vi "Voltage - Continuous Input_0317.vi"() -> ()   [LabVIEW 2021]
doc: "This example demonstrates how to continuously acquire buffered voltage measurements using a DAQmx device.\n\nFor instructions on how to connect your signals to the DAQ device, refer to your device documentation."
uses:
  <vilib>/Utility/error.llb/DialogType.ctl
  <vilib>/DAQmx/read.llb/DAQmx Read (Analog 1D Wfm NChan NSamp).vi
  <vilib>/DAQmx/create/channels.llb/DAQmx Create Channel (AI-Voltage-Basic).vi
  <vilib>/DAQmx/configure/timing.llb/DAQmx Timing (Sample Clock).vi
  <vilib>/DAQmx/configure/task.llb/DAQmx Configure Logging (TDMS).vi
  <vilib>/DAQmx/configure/trigger.llb/DAQmx Start Trigger (Digital Edge).vi
  <vilib>/DAQmx/configure/trigger.llb/DAQmx Start Trigger (Time).vi
  <vilib>/DAQmx/configure/trigger.llb/DAQmx Start Trigger (Analog Edge).vi
  <vilib>/DAQmx/miscellaneous.llb/DAQmx Fill In Error Info.vi
  <resource>/objmgr/daqmx.rc
panel:
  in  "Physical Channel 2":tag="Dev1/ai0"
  in  "Min Voltage 2":dbl=-5.0
  in  "Max Voltage 2":dbl=5.0
  in  "Trigger Type":T1(tab)
  in  "Digital Start Trigger Edge":i32(ring)=10280 caption="Edge" items=["Rising"=10280, "Falling"=10171]
  in  "Digital Start Trigger Source":tag="/Dev1/PFI0" caption="Source"
  in  "Digital Pause Trigger Pause When":i32(ring)=10192 caption="Pause When" items=["High"=10192, "Low"=10214]
  in  "Digital Pause Trigger Source":tag="/Dev1/PFI0" caption="Source"
  in  "Analog Start Trigger Level":dbl caption="Level" format="%0.2f"
  in  "Analog Start Trigger Hysteresis":dbl caption="Hysteresis" format="%.2f"
  in  "Analog Start Trigger Slope":i32(ring)=10280 caption="Slope" items=["Rising"=10280, "Falling"=10171]
  in  "Analog Start Trigger Source":string="APFI0" caption="Source"
  in  "Analog Pause Trigger Source":string="APFI0" caption="Source"
  in  "Analog Pause Trigger Pause When":i32(ring)=10093 caption="Pause When" items=["Above Level"=10093, "Below Level"=10107]
  in  "Analog Pause Trigger Level":dbl caption="Level" format="%.2f"
  in  "When":timestamp
  in  "Select Time\nManually":bool
  in  "Stop":bool
  out "Waveform Graph":waveform(dbl)[](graph)
  in  "TDMS File Path":path
  in  "Number of Samples":i32=100
  in  "Sample Rate":dbl=1000.0
  in  "Sample Clock Source":tag="OnboardClock"
  in  "Terminal Configuration":i32(ring)=-1 items=["default"=-1, "RSE"=10083, "NRSE"=10078, "Differential"=10106, "Pseudodifferential"=12529]
  in  "Max Voltage":dbl=5.0
  in  "Min Voltage":dbl=-5.0
  in  "Physical Channel":tag="Dev1/ai0"
  out "Actual Sample Rate":dbl=1000.0 format="%0.2f"
  in  "Logging Mode":i32(ring)=10231 items=["Off"=10231, "Log and Read"=15842]
  # "Channel Settings"
  # "Acquired Data"
  # "Timing Settings"
  # "Trigger Settings"
  # "Logging Settings"
  # "To enable triggers, select a tab above, and configure the settings.\n\nNot all hardware supports all trigger types. Refer to your device documentation for more information."
  # "This trigger type is not supported in continuous sample timing. \n\nRefer to your device documentation for more information on which triggers are supported."
  # "This trigger type is not supported in continuous sample timing. \n\nRefer to your device documentation for more information on which triggers are supported."
  # "If time is not manually set, task will begin after 10 seconds"
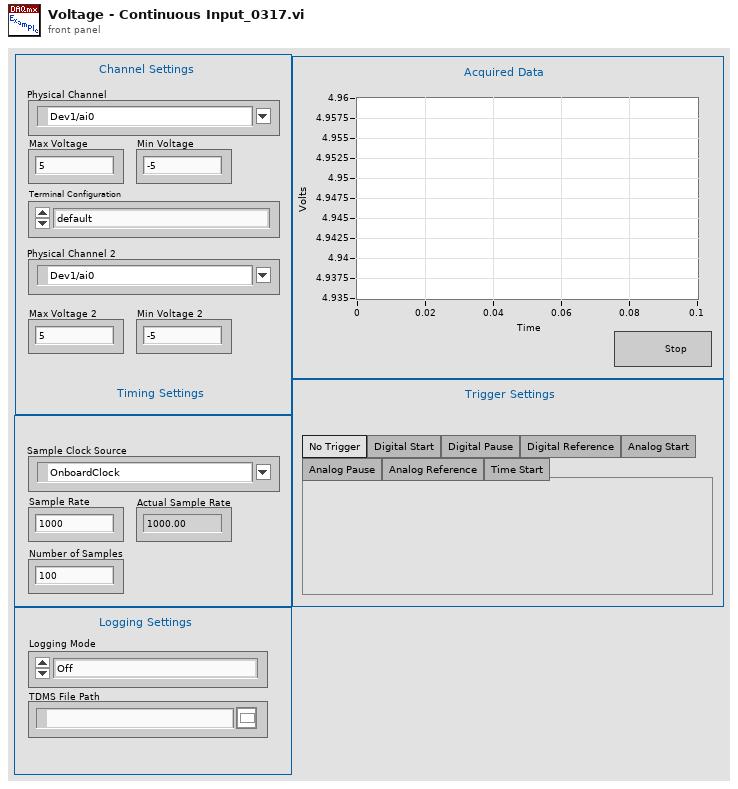
[diagram p1: front panel]
types:
  T1 = enum32{"No Trigger", "Digital Start", "Digital Pause", "Digital Reference", "Analog Start", "Analog Pause", "Analog Reference", "Time Start"}
  T2 = typedef "DialogType.ctl" = u16
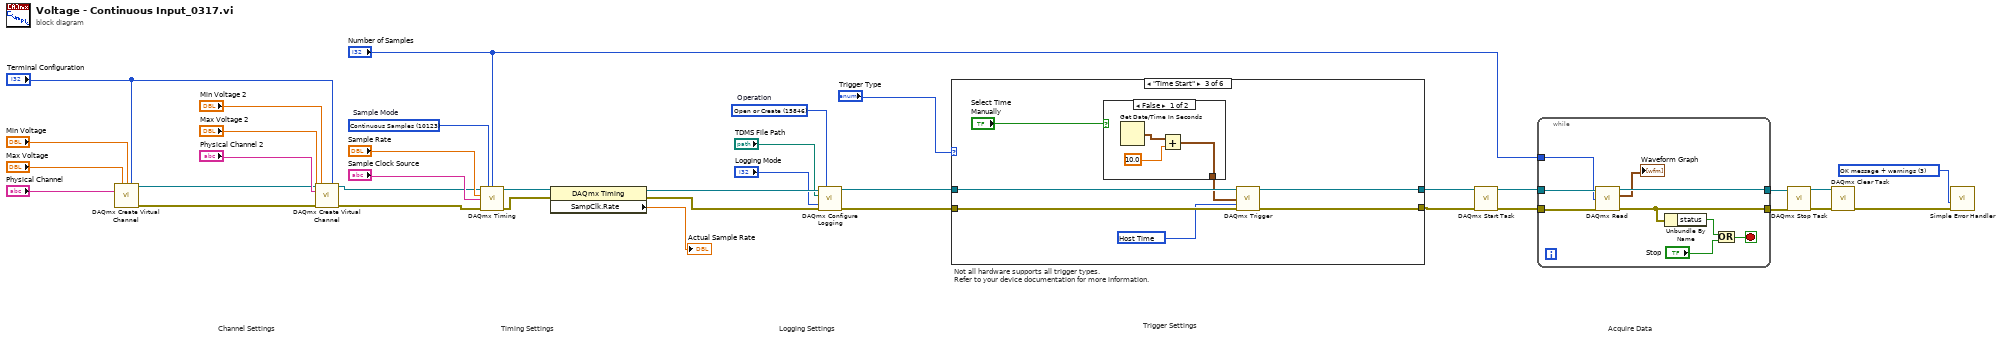
[diagram p0: block diagram]
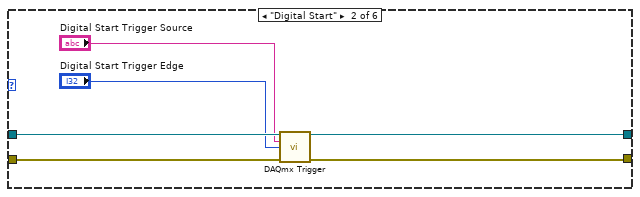
[diagram p3: hidden frame]
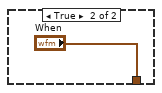
[diagram p4: hidden frame]
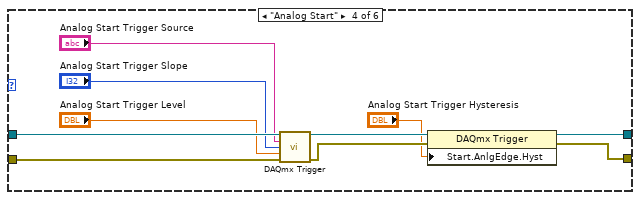
[diagram p5: hidden frame]
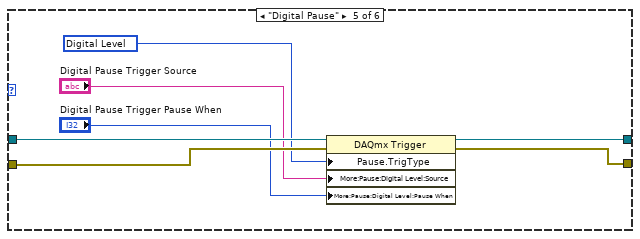
[diagram p6: hidden frame]
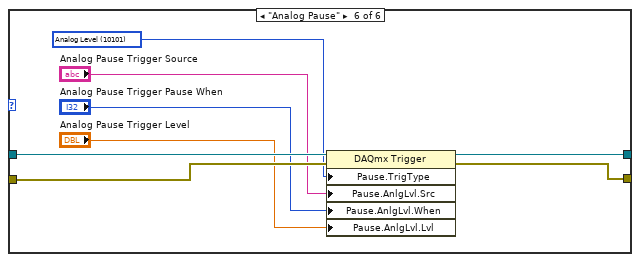
[diagram p7: hidden frame]
diagram:
  w14 = T2 3 items=["no dialog", "OK message", "continue or stop message", "OK message + warnings", "continue/stop + warnings"] ("type of dialog (OK msg:1)")
  w31 = 15846 items=["Open"=10437, "Open or Create"=15846, "Create or Replace"=15847, "Create"=15848]  # Operation
  w34 = 10123 items=["Finite Samples"=10178, "Continuous Samples"=10123, "Hardware Timed Single Point"=12522]  # Sample Mode
  # "Trigger Settings"
  # "Not all hardware supports all trigger types.\nRefer to your device documentation for more information."
  # "Acquire Data"
  # "Timing Settings"
  # "Channel Settings"
  # "Logging Settings"
  n1 = call-poly <vilib>:"DAQmx Create Virtual Channel.vi"("maximum value"="Max Voltage", "minimum value"="Min Voltage", "input terminal configuration"="Terminal Configuration", "physical channels"="Physical Channel") -> ("task out"=w5:refnum<k21>, "error out"=w4:errorcluster)  [unwired: 10 in]
  n2 = call-poly <vilib>:"DAQmx Create Virtual Channel.vi"("task in"=w5, "maximum value"="Max Voltage 2", "minimum value"="Min Voltage 2", "input terminal configuration"="Terminal Configuration", "physical channels"="Physical Channel 2", "error in"=w4) -> ("task out"=w3:refnum<k21>, "error out"=w2:errorcluster)  [unwired: 8 in]
  n3 = call-poly <vilib>:"DAQmx Timing.vi"("task/channels in"=w3, "sample mode"=w34, "samples per channel"="Number of Samples", "rate"="Sample Rate", "source"="Sample Clock Source", "error in"=w2) -> ("task out"=w36:refnum<k21>, "error out"=w35:errorcluster)  [unwired: 8 in]
  n4 = property class="DAQmx Timing"(reference=w36, error in=w35) -> (reference out=w33:refnum<k21>, error out=w32:errorcluster, "SampClk.Rate"=→"Actual Sample Rate":dbl)
  n5 = call-poly <vilib>:"DAQmx Configure Logging.vi"("task/channels in"=w33, "operation"=w31, "file path"="TDMS File Path", "logging mode"="Logging Mode", "error in"=w32) -> ("task out"=w12:refnum<k21>, "error out"=w11:errorcluster)  [unwired: 9 in]
  n6 = case shown="\"Time Start\"" "Trigger Type" {
    tunnel: w12 -> [w38 w44 w51 w65 w72 w80]
    tunnel: w11 -> [w37 w43 w50 w64 w69 w77]
    tunnel: [w38 w42 w49 w62 w71 w79] -> w9
    tunnel: [w37 w41 w48 w61 w70 w78] -> w10
    frame "No Trigger", Default {
    }
    frame "Digital Start" {
      n7 = call-poly <vilib>:"DAQmx Trigger.vi"("task/channels in"=w44, "source"="Digital Start Trigger Source", "edge"="Digital Start Trigger Edge", "error in"=w43) -> ("task out"=w42:refnum<k21>, "error out"=w41:errorcluster)  [unwired: 10 in]
    }
    frame "Time Start" {
      w47 = 16126 items=["Host Time"=16126, "I/O Device Time"=16127] ("timescale")
      n8 = case shown="False" "Select Time\nManually" {
        tunnel: [w52 "When"] -> w45
        frame False {
          n9 = Get Date/Time In Seconds() -> (seconds since 1Jan1904=w54:timestamp)
          n10 = Add(x=w54, y=10.0) -> (x+y=w52:timestamp)
        }
        frame True {
        }
      }
      n11 = call-poly <vilib>:"DAQmx Trigger.vi"("task/channels in"=w51, "when"=w45, "timescale"=w47, "error in"=w50) -> ("task out"=w49:refnum<k21>, "error out"=w48:errorcluster)  [unwired: 10 in]
    }
    frame "Analog Start" {
      n12 = call-poly <vilib>:"DAQmx Trigger.vi"("task/channels in"=w65, "source"="Analog Start Trigger Source", "slope"="Analog Start Trigger Slope", "level"="Analog Start Trigger Level", "error in"=w64) -> ("task out"=w60:refnum<k21>, "error out"=w59:errorcluster)  [unwired: 9 in]
      n13 = property class="DAQmx Trigger"(reference=w60, error in=w59, "Start.AnlgEdge.Hyst"="Analog Start Trigger Hysteresis") -> (reference out=w62:refnum<k21>, error out=w61:errorcluster)
    }
    frame "Digital Pause" {
      w68 = 10152 items=["Analog Level"=10101, "Analog Window"=10103, "Digital Level"=10152, "Digital Pattern"=10398, "None"=10230] ("Pause.TrigType")
      n14 = property class="DAQmx Trigger"(reference=w72, error in=w69, "Pause.TrigType"=w68, "More:Pause:Digital Level:Source"="Digital Pause Trigger Source", "More:Pause:Digital Level:Pause When"="Digital Pause Trigger Pause When") -> (reference out=w71:refnum<k21>, error out=w70:errorcluster)
    }
    frame "Analog Pause" {
      w76 = 10101 items=["Analog Level"=10101, "Analog Window"=10103, "Digital Level"=10152, "Digital Pattern"=10398, "None"=10230] ("Pause.TrigType")
      n15 = property class="DAQmx Trigger"(reference=w80, error in=w77, "Pause.TrigType"=w76, "Pause.AnlgLvl.Src"="Analog Pause Trigger Source", "Pause.AnlgLvl.When"="Analog Pause Trigger Pause When", "Pause.AnlgLvl.Lvl"="Analog Pause Trigger Level") -> (reference out=w79:refnum<k21>, error out=w78:errorcluster)
    }
  }
  n16 = call <vilib>:"DAQmx Start Task.vi"("task/channels in"=w9, "error in"=w10) -> ("task out"=w30:refnum<k21>, "error out"=w29:errorcluster)  [unwired: 12 in]
  n17 = while {
    tunnel: w30 -> [w89]
    tunnel: w29 -> [w88]
    tunnel: [w87] -> w18
    tunnel: [w84] -> w17
    tunnel: "Number of Samples" -> [w81]
    stop <- w82 stop-if-true
    n18 = call-poly <vilib>:"DAQmx Read.vi"("task/channels in"=w89, "number of samples per channel"=w81, "error in"=w88) -> ("task out"=w87:refnum<k21>, "data"=→"Waveform Graph":waveform(dbl)[], "error out"=w84:errorcluster)  [unwired: 10 in]
    n19 = Unbundle By Name(w84) -> ("status"=w83:bool)
    n20 = Or(x=w83, y="Stop") -> (x .or. y?=w82:bool)
  }
  n21 = call <vilib>:"DAQmx Stop Task.vi"("task/channels in"=w18, "error in"=w17) -> ("task out"=w15:refnum<k21>, "error out"=w16:errorcluster)  [unwired: 12 in]
  n22 = call <vilib>:"DAQmx Clear Task.vi"("task in"=w15, "error in"=w16) -> ("error out"=w28:errorcluster)  [unwired: 13 in]
  n23 = call <vilib>:"Simple Error Handler.vi"("type of dialog (OK msg:1)"=w14, "error in (no error)"=w28) -> ()  [unwired: 3 in, 5 out]
